vi "PRIOR_Initialize.vi"() -> (0 "错误输出":errorcluster, 3 "VISA资源名称输出":refnum<visa-resource-name>)   [LabVIEW 2018]
uses:
  <vilib>/Instr/_visa.llb/VISA Configure Serial Port (Instr).vi
panel:
  in  "error in (no error)":errorcluster caption="错误输入（无错误）"
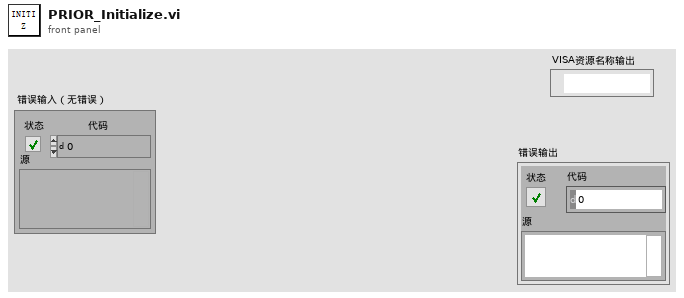
[diagram p1: front panel]
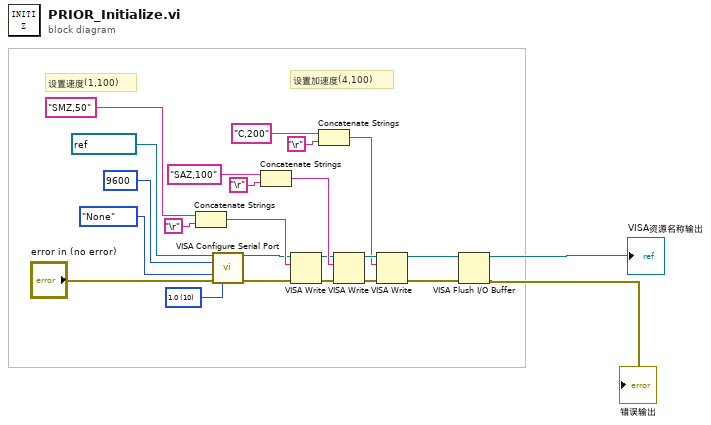
[diagram p0: block diagram]
diagram:
  w21 = u16 10 items=["1.0"=10, "1.5"=15, "2.0"=20] ("停止位 (10: 1位)")
  # "设置加速度(4,100)"
  # "设置速度(1,100)"
  n1 = Concatenate Strings("SMZ,50" ("写入缓冲区"), "\r") -> (w18:string)
  n2 = call-poly "VISA Configure Serial Port"("VISA resource name"=refnum<visa-resource-name> "COM9" ("VISA资源名称"), "baud rate (9600)"=u32 9600 ("波特率(9600)"), "parity (0:none)"=enum16{"None", "Odd", "Even", "Mark", "Space"}."None" ("校验（无）"), "error in (no error)"="error in (no error)", "stop bits (10: 1 bit)"=w21) -> ("VISA resource name out"=w16:refnum<visa-resource-name>, "error out"=w15:errorcluster)  [unwired: 9 in]
  n3 = Concatenate Strings("SAZ,100" ("写入缓冲区"), "\r") -> (w13:string)
  n4 = VISA Write ("VISA写入")(VISA resource name=w16, write buffer=w18, error in (no error)=w15) -> (VISA resource name out=w11:refnum<visa-resource-name>, error out=w10:errorcluster)  [unwired: 1 out]
  n5 = Concatenate Strings("C,200" ("写入缓冲区"), "\r") -> (w5:string)
  n6 = VISA Write ("VISA写入")(VISA resource name=w11, write buffer=w13, error in (no error)=w10) -> (VISA resource name out=w9:refnum<visa-resource-name>, error out=w8:errorcluster)  [unwired: 1 out]
  n7 = VISA Write ("VISA写入")(VISA resource name=w9, write buffer=w5, error in (no error)=w8) -> (VISA resource name out=w4:refnum<visa-resource-name>, error out=w3:errorcluster)  [unwired: 1 out]
  n8 = VISA Flush I/O Buffer(VISA resource name=w4, error in (no error)=w3) -> (VISA resource name out=→"VISA资源名称输出":refnum<visa-resource-name>, error out=→"错误输出":errorcluster)  [unwired: 1 in]
